vi "TWM Client Send Packet.vi"(7 "end of packet key":string="TWM:command:EndOfPacket", 8 "error in":errorcluster, 10 "command string":string, 11 "handle":i32) -> (0 "error out":errorcluster, 3 "handle out":i32)   [LabVIEW 2013]
doc: "Write command packet to TWM server."
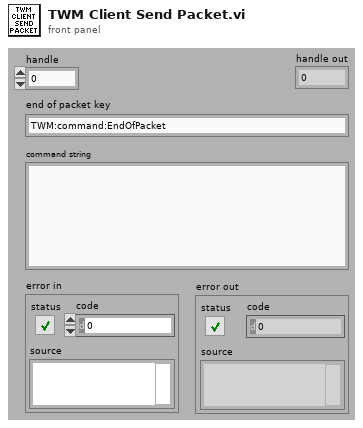
[diagram p1: front panel]
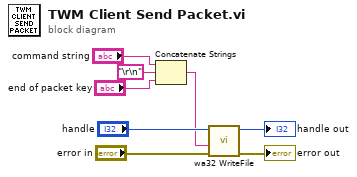
[diagram p0: block diagram]
diagram:
  n1 = Concatenate Strings("command string", "\r\n", "end of packet key") -> (w3:string)
  n2 = call "wa32 WriteFile.vi"("error in"="error in", "string data (empty)"=w3, "handle"="handle") -> ("error out"=→"error out":errorcluster, "handle out"=→"handle out":i32)  [unwired: 6 in, 1 out]
